vi "GFITS_LibGetExtensions.vi"(8 "error in (no error)":errorcluster) -> (0 "error out":errorcluster, 1 "array out":i32[](array[numeric]), 2 "num extensions":i32, 3 "max_ext":i32, 4 "discard":bool[](array[boolean]))   [LabVIEW 2016]
uses:
  c/lib/libgfits.so
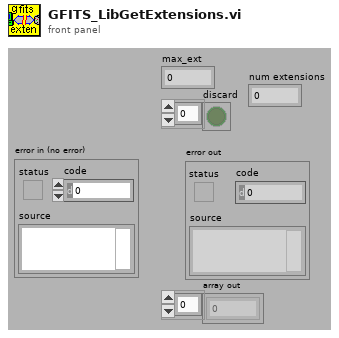
[diagram p1: front panel]
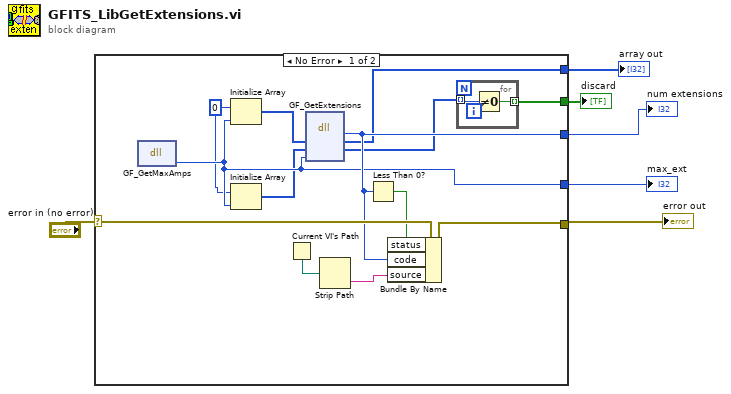
[diagram p0: block diagram]
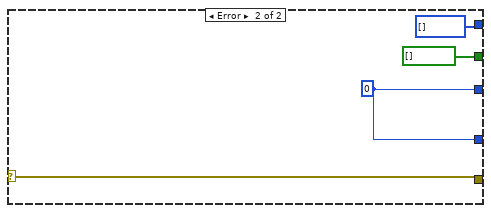
[diagram p2: hidden frame]
diagram:
  n1 = case shown="No Error" "error in (no error)" {
    selector: "error in (no error)" -> [w19 w25]
    tunnel: [w17 w24] -> w6
    tunnel: [w14 w25] -> w4
    tunnel: [w12 w24] -> w3
    tunnel: [w8 i32[] [] ("array")] -> w2
    tunnel: [w7 bool[] []] -> w1
    frame No Error {
      w11 = 0 ("element")
      n2 = dll-call lib="home/simager/panview/PAN/Modules/GFITS/private/c/lib/libgfits.so" fn="GF_GetMaxAmps"() -> ("return type"=w12:i32)  [unwired: 3 in, 2 out]
      n3 = Initialize Array(w11, w12) -> (w13:i32[])
      n4 = Initialize Array(w11, w12) -> (w10:i32[])
      n5 = Current VI's Path() -> (path=w16:path)
      n6 = dll-call lib="home/simager/panview/PAN/Modules/GFITS/private/c/lib/libgfits.so" fn="GF_GetExtensions"("array"=w13, "discard"=w10, "num_elements"=w12) -> ("return type"=w17:i32, "array"=w8:i32[], "discard"=w9:i32[])  [unwired: 4 in, 2 out]
      n7 = Strip Path(path=w16) -> (name=w15:string)  [unwired: 1 out]
      n8 = Less Than 0?(x=w17) -> (x < 0?=w18:bool)
      n9 = Bundle By Name(cluster=w19, "status"=w18, "code"=w17, "source"=w15) -> (w14:errorcluster)
      n10 = for {
        tunnel: w9 -> [w21] mode=indexing
        tunnel: [w20] -> w7 mode=indexing
        n11 = Not Equal To 0?(x=w21) -> (x != 0?=w20:bool)
      }
    }
    frame Error {
      w24 = 0
    }
  }
  "num extensions" <- w6
  "error out" <- w4
  "max_ext" <- w3
  "array out" <- w2
  "discard" <- w1
